vi "Wave-Parse EPL Chunk.vi"(8 "error in (no error)":errorcluster, 10 "chunk info":T2, 11 "refnum":refnum<file>) -> (0 "error out":errorcluster, 2 "EPL Variables":T1[](array[typedef]), 3 "refnum out":refnum<file>)   [LabVIEW 2020]
uses:
  Wave-Chunk Info.ctl
  Wave-EPL Chunk Variable.ctl
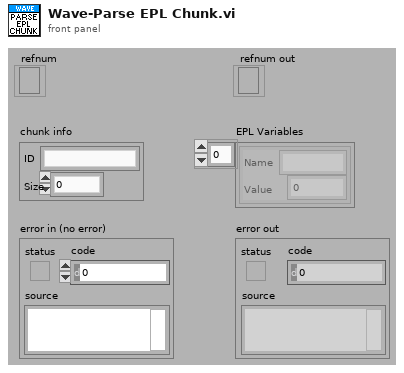
[diagram p1: front panel]
types:
  T1 = typedef "Wave-EPL Chunk Variable.ctl" = cluster{"Name":string, "Value":dbl}
  T2 = typedef "Wave-Chunk Info.ctl" = cluster{"ID":string, "Size":u32}
  T3 = enum16{"big-endian, network order", "native, host order", "little-endian"}
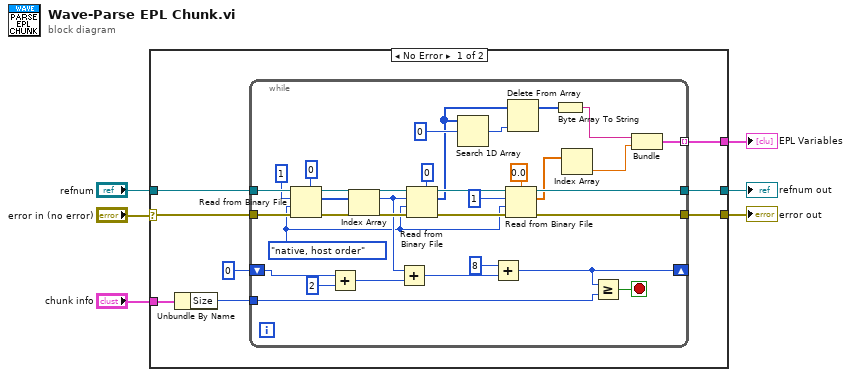
[diagram p0: block diagram]
diagram:
  n1 = case shown="No Error" "error in (no error)" {
    selector: "error in (no error)" -> [w13 w47]
    tunnel: "refnum" -> [w14 w48]
    tunnel: [w10 w48] -> w5
    tunnel: [w9 w47] -> w3
    tunnel: "chunk info" -> [w12 _]
    tunnel: [w7 _] -> w1
    frame No Error {
      n2 = Unbundle By Name(w12) -> ("Size"=w11:u32)
      n3 = while {
        tunnel: w14 -> [w46]
        tunnel: w13 -> [w44]
        tunnel: w11 -> [w28]
        tunnel: [w34] -> w10
        tunnel: [w36] -> w9
        shift-right: [w29] -> _
        shift-left: 0 -> [w25]
        tunnel: [w20] -> w7 mode=indexing
        stop <- w27 stop-if-true
        w33 = T3."native, host order" ("byte order (0:big-endian, network order)")
        n4 = Read from Binary File(5:u16 0, 8:w44, 9:w33, 10:1, 11:w46) -> (0:w42:errorcluster, 2:w40:u16[], 3:w41:refnum<file>)  [unwired: 1 in, 1 out]
        n5 = Add(x=w25, y=2) -> (x+y=w24:i32)
        n6 = Index Array(array=w40) -> (element=w38:u16)  [unwired: 1 in]
        n7 = Add(x=w38, y=w24) -> (x+y=w31:i32)
        n8 = Read from Binary File(5:u8 0, 8:w42, 9:w33, 10:w38, 11:w41) -> (0:w37:errorcluster, 2:w15:u8[], 3:w35:refnum<file>)  [unwired: 1 in, 1 out]
        n9 = Search 1D Array(1D array=w15, element=u8 0) -> (index of element=w18:i32)  [unwired: 1 in]
        n10 = Add(x=8, y=w31) -> (x+y=w29:i32)
        n11 = Read from Binary File(5:0.0, 8:w37, 9:w33, 10:1 ("count (1)"), 11:w35) -> (0:w36:errorcluster, 2:w26:dbl[], 3:w34:refnum<file>)  [unwired: 1 in, 1 out]
        n12 = Delete From Array(array=w15, index=w18) -> (array with subset deleted=w16:u8[])  [unwired: 1 in, 1 out]
        n13 = Byte Array To String(unsigned byte array=w16) -> (string=w17:string)
        n14 = Index Array(array=w26) -> (element=w21:dbl)  [unwired: 1 in]
        n15 = Greater Or Equal?(x=w29, y=w28) -> (x >= y?=w27:bool)
        n16 = Bundle("string"=w17, w21) -> (w20:cluster{"string":string, dbl})  [unwired: 1 in]
      }
    }
    frame Error {
    }
  }
  "error out" <- w3
  "refnum out" <- w5
  "EPL Variables" <- w1
